vi "Prog3.vi"() -> ()   [LabVIEW 2021]
panel:
  out "concatenated string 5":string
  out "concatenated string 4":string
  out "concatenated string 3":string
  out "concatenated string 2":string
  out "concatenated string":string
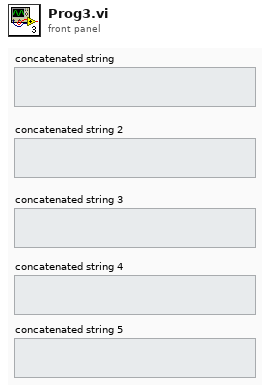
[diagram p1: front panel]
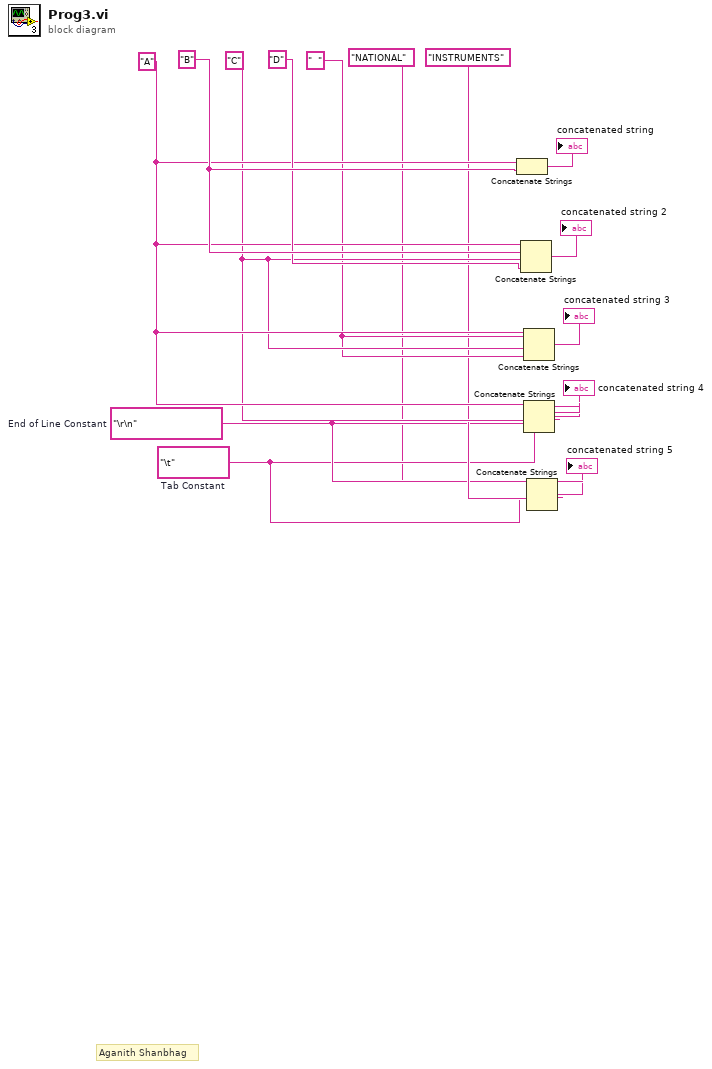
[diagram p0: block diagram]
diagram:
  w8 = "\r\n"  # End of Line Constant
  w7 = "\t"  # Tab Constant
  w10 = "  "
  w11 = "C"
  w14 = "B"
  w12 = "A"
  # "Aganith Shanbhag"
  n1 = Concatenate Strings "Concatenate Strings"(w12, w14) -> (→"concatenated string":string)
  n2 = Concatenate Strings "Concatenate Strings"(w12, w14, w11, "D") -> (→"concatenated string 2":string)
  n3 = Concatenate Strings "Concatenate Strings"(w12, w10, w11, w10) -> (→"concatenated string 3":string)
  n4 = Concatenate Strings "Concatenate Strings"(w12, w8, w11, w7) -> (→"concatenated string 4":string)
  n5 = Concatenate Strings "Concatenate Strings"("NATIONAL", w8, "INSTRUMENTS", w7) -> (→"concatenated string 5":string)
